vi "FSM Editor Write.vi"(4 "error in (no error)":errorcluster, 5 "Value":bool, 6 "Container State":T5, 7 "Display State In":T1) -> (0 "error out":errorcluster, 3 "Display State Out":T1)   [LabVIEW 2015, in "FSM Editor.xctl"]
uses:
  FSM Editor.xctl
  <vilib>/_xctls/Container State.ctl
  <vilib>/_xctls/XControlSupport.lvlib
  NodeAdded.ctl
  Events.ctl
  <vilib>/Utility/miscctls.llb/LVPoint32TypeDef.ctl
  Drag Mode.ctl
  Classes/FSM.Port/FSM.Port.lvclass
  State.vi
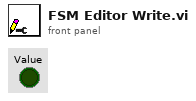
[diagram p1: front panel]
types:
  T1 = typedef "FSM Editor.xctl/State.vi" = cluster{"snap":bool, "default name":string, "dragStartPoint":T2, "dragMode":T3, "gridsize":dbl, "selectRect":cluster{"left":i16, "top":i16, "right":i16, "bottom":i16}, "events":string[], "cs+/cs-":bool, "insertEdgeAt":string, "insertingEdge":bool, "activePort":refnum<class "FSM.Port.lvclass">, "sourcePort":refnum<class "FSM.Port.lvclass">, "insertionEnd":cluster{"x":i16, "y":i16}, "insertEdgeSpec":string, "nodeIndex":i32, "Events":T4, "action":string}
  T2 = typedef "LVPoint32TypeDef.ctl" = cluster{"Horizontal":i32, "Vertical":i32}
  T3 = typedef "Drag Mode.ctl" = enum16{"Off", "NodePending", "Nodes", "Pan", "Select", "EdgeInsertion", "EdgePoint", "EdgeLabel"}
  T4 = typedef "FSM Editor.xctl/Events.ctl" = cluster{"NodeAdded":refnum<user-event>}
  T5 = typedef "XControlSupport.lvlib/Container State.ctl" = cluster{"Indicator?":bool, "Run Mode?":bool, " Refnum":refnum<vi>}
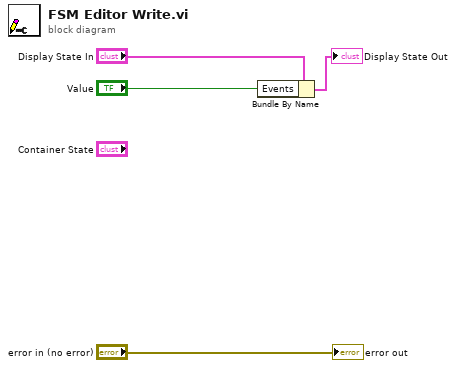
[diagram p0: block diagram]
diagram:
  n1 = Bundle By Name(cluster="Display State In", "Events"="Value") -> (→"Display State Out":T1)
  "error out" <- "error in (no error)"
